vi "SaveData.vi"(5 "Save":bool, 7 "# Sample Points":i32=4096, 11 "Data":dbl[](array[numeric])) -> ()   [LabVIEW 2017]
uses:
  <vilib>/Utility/file.llb/Write Delimited Spreadsheet (DBL).vi
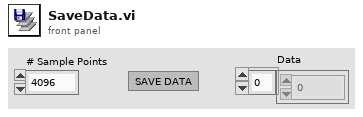
[diagram p1: front panel]
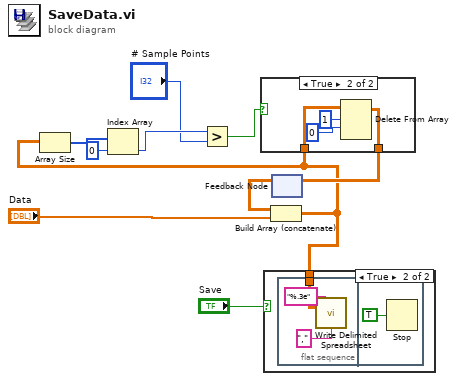
[diagram p0: block diagram]
diagram:
  n1 = feedback #1() -> (w10:dbl[][])  [unwired: 1 in]
  n2 = Build Array (concatenate)(w10, "Data") -> (w2:dbl[][])
  n3 = Array Size(array=w2) -> (size(s)=w9:i32[])
  n4 = Index Array(array=w9, index=0) -> (element=w7:i32)
  n5 = Greater?(x=w7, y="# Sample Points") -> (0:w5:bool)
  n6 = case shown="True" w5 {
    tunnel: w2 -> [w11 w15]
    tunnel: [w11 w14] -> w4
    frame False {
    }
    frame True {
      n7 = Delete From Array(array=w15, length=1, index (row)=0) -> (array with subset deleted=w14:dbl[][])  [unwired: 1 in, 1 out]
    }
  }
  n8 = case shown="True" "Save" {
    tunnel: w2 -> [_ w16]
    frame False {
    }
    frame True {
      n9 = flat-sequence {
        tunnel: w16 -> [w19]
        frame #0 {
          n10 = call-poly <vilib>:"Write Delimited Spreadsheet.vi"("format (%.3f)"="%.3e", "2D data"=w19, "delimiter (\\t)"="," ("delimiter (\\t)")) -> ()  [unwired: 11 in, 2 out]
        }
        frame #1 {
          n11 = Stop(stop? (T)=TRUE) -> ()
        }
      }
    }
  }
  n12 = feedback-in #1(w4) -> ()
